vi "Target Get Prosthesis Parameters.vi"() -> (1 "Lever Arm Polynomial":dbl[](array[numeric]), 3 "Spring Polynomial":dbl[](array[numeric]))   [LabVIEW 2018, in "COBRA Prosthesis Model Library.lvlib"]
uses:
  COBRA Prosthesis Model Library.lvlib
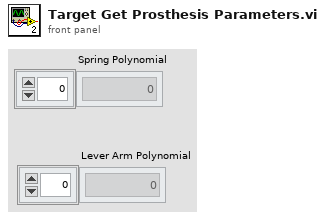
[diagram p1: front panel]
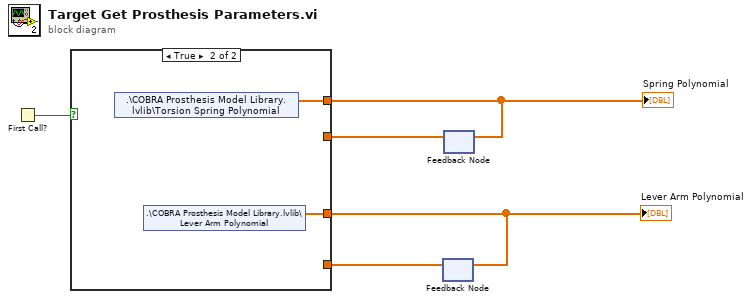
[diagram p0: block diagram]
diagram:
  n1 = First Call?() -> (First Call?: T/F=w5:bool)
  n2 = feedback #1() -> (w1:dbl[])  [unwired: 1 in]
  n3 = feedback #2() -> (w3:dbl[])  [unwired: 1 in]
  n4 = case shown="True" w5 {
    tunnel: [w7 w9] -> w4
    tunnel: w3 -> [w7 _]
    tunnel: [w6 w8] -> w2
    tunnel: w1 -> [w6 _]
    frame False {
    }
    frame True {
      n5 = shared-variable ".\\COBRA Prosthesis Model Library.lvlib\\Torsion Spring Polynomial"() -> (w9:dbl[])  [unwired: 1 in, 1 out]
      n6 = shared-variable ".\\COBRA Prosthesis Model Library.lvlib\\Lever Arm Polynomial"() -> (w8:dbl[])  [unwired: 1 in, 1 out]
    }
  }
  "Lever Arm Polynomial" <- w2
  "Spring Polynomial" <- w4
  n7 = feedback-in #1(w2) -> ()
  n8 = feedback-in #2(w4) -> ()
